vi "Color Grabber.vi"(10 "control-level":string, 11 "Material-Scheme in":refnum<class "Material-Scheme.lvclass">) -> (0 "onSurface":u32, 1 "surface":u32, 2 "onColor":u32, 3 "color":u32, 4 "colorContainer":u32, 5 "outline":u32, 6 "onColorContainer":u32)   [LabVIEW 2021, in "TSC Material Theme.lvlib" / "Material-Scheme.lvclass"]
doc: "get the colorset for the application and the color-level\n\n<b>Code Developed By:</b>\nTechnology Service Corporation\nwww.tsc.com/atcs\n\nDeveloper:\nDaniel Coons"
uses:
  Material-Scheme.lvclass
  Material-Scheme.lvclass/Material-Scheme.ctl
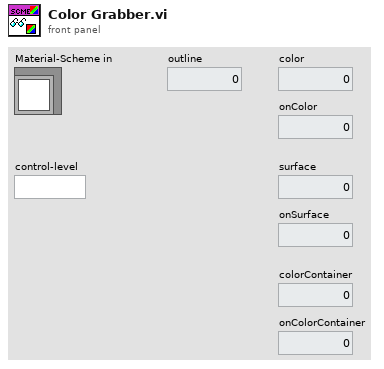
[diagram p1: front panel]
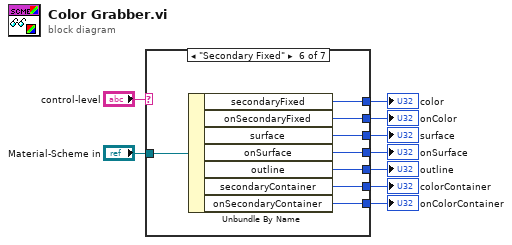
[diagram p0: block diagram]
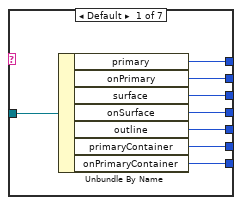
[diagram p2: hidden frame]
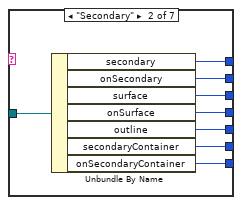
[diagram p3: hidden frame]
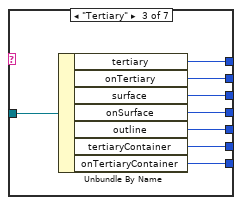
[diagram p4: hidden frame]
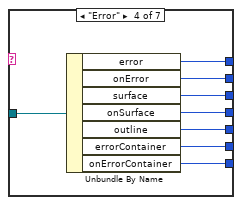
[diagram p5: hidden frame]
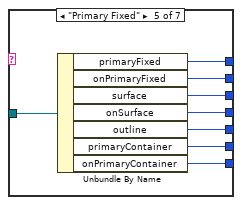
[diagram p6: hidden frame]
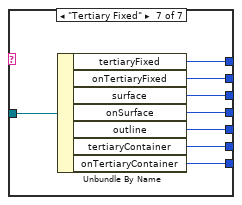
[diagram p7: hidden frame]
diagram:
  n1 = case shown="\"Secondary Fixed\"" "control-level" {
    tunnel: [w17 w25 w33 w41 w49 w57 w65] -> w5
    tunnel: "Material-Scheme in" -> [w16 w24 w32 w40 w48 w56 w64]
    tunnel: [w15 w23 w31 w39 w47 w55 w63] -> w7
    tunnel: [w13 w21 w29 w37 w45 w53 w61] -> w4
    tunnel: [w14 w22 w30 w38 w46 w54 w62] -> w8
    tunnel: [w12 w20 w28 w36 w44 w52 w60] -> w3
    tunnel: [w11 w18 w26 w34 w42 w50 w58] -> w2
    tunnel: [w10 w19 w27 w35 w43 w51 w59] -> w1
    frame Default {
      n2 = Unbundle By Name(w16) -> ("primary"=w17:u32, "onPrimary"=w13:u32, "surface"=w15:u32, "onSurface"=w14:u32, "outline"=w12:u32, "primaryContainer"=w11:u32, "onPrimaryContainer"=w10:u32)
    }
    frame "Secondary" {
      n3 = Unbundle By Name(w24) -> ("secondary"=w25:u32, "onSecondary"=w21:u32, "surface"=w23:u32, "onSurface"=w22:u32, "outline"=w20:u32, "secondaryContainer"=w18:u32, "onSecondaryContainer"=w19:u32)
    }
    frame "Tertiary" {
      n4 = Unbundle By Name(w32) -> ("tertiary"=w33:u32, "onTertiary"=w29:u32, "surface"=w31:u32, "onSurface"=w30:u32, "outline"=w28:u32, "tertiaryContainer"=w26:u32, "onTertiaryContainer"=w27:u32)
    }
    frame "Error" {
      n5 = Unbundle By Name(w40) -> ("error"=w41:u32, "onError"=w37:u32, "surface"=w39:u32, "onSurface"=w38:u32, "outline"=w36:u32, "errorContainer"=w34:u32, "onErrorContainer"=w35:u32)
    }
    frame "Primary Fixed" {
      n6 = Unbundle By Name(w48) -> ("primaryFixed"=w49:u32, "onPrimaryFixed"=w45:u32, "surface"=w47:u32, "onSurface"=w46:u32, "outline"=w44:u32, "primaryContainer"=w42:u32, "onPrimaryContainer"=w43:u32)
    }
    frame "Secondary Fixed" {
      n7 = Unbundle By Name(w56) -> ("secondaryFixed"=w57:u32, "onSecondaryFixed"=w53:u32, "surface"=w55:u32, "onSurface"=w54:u32, "outline"=w52:u32, "secondaryContainer"=w50:u32, "onSecondaryContainer"=w51:u32)
    }
    frame "Tertiary Fixed" {
      n8 = Unbundle By Name(w64) -> ("tertiaryFixed"=w65:u32, "onTertiaryFixed"=w61:u32, "surface"=w63:u32, "onSurface"=w62:u32, "outline"=w60:u32, "tertiaryContainer"=w58:u32, "onTertiaryContainer"=w59:u32)
    }
  }
  "onSurface" <- w8
  "onColor" <- w4
  "surface" <- w7
  "color" <- w5
  "outline" <- w3
  "onColorContainer" <- w1
  "colorContainer" <- w2
